vi "FPGA_Looped_PC.vi"() -> (0 "Chassis Temp History":i16[](array[numeric]), 3 "Chassis Temperature":i16)   [LabVIEW 2020]
uses:
  UIcontrol.ctl
  <vilib>/rvi/interface/RandomDataEmulation/nirviRandomDataOpen.vi
  <vilib>/rvi/interface/common/niFpgaCacheSessionInfoDynamic.vi
  <vilib>/Utility/error.llb/Error Cluster From Error Code.vi
  <vilib>/rvi/errors/niLvFpgaAdjustHostInterfaceError.vi
  <vilib>/rvi/interface/nirviOpenFPGA/nirviOpenFPGA.xnode
  FPGA_Temp.vi
  <vilib>/rvi/interface/nirviReadWriteControl/nirviReadWriteControl.xnode
  NiFpgaLv.dll
  <vilib>/rvi/interface/Simulation/niFpgaSimulationCallBeginRW.vi
panel:
  in  "cRIO Shutdown":bool
  in  "cRIO Save Data":bool
  in  "cRIO Start":bool
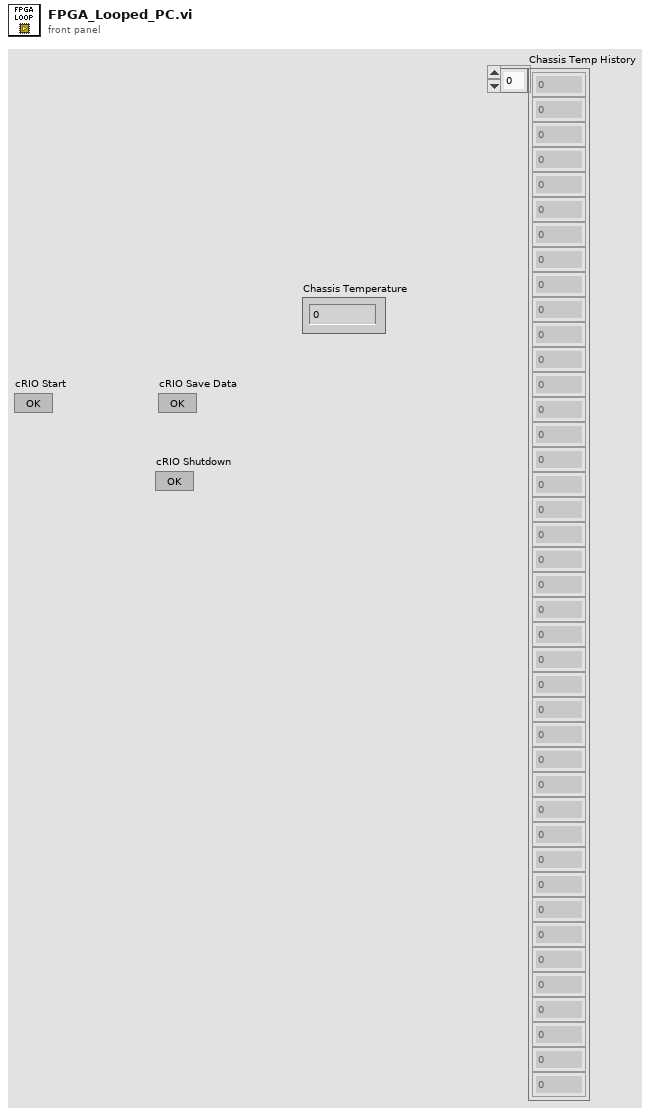
[diagram p1: front panel]
types:
  T1 = typedef "UIcontrol.ctl" = enum16{"Start", "Save Data", "Shutdown"}
  T2 = enum16{"open", "replace", "create", "open or create", "replace or create", "replace or create with confirmation"}
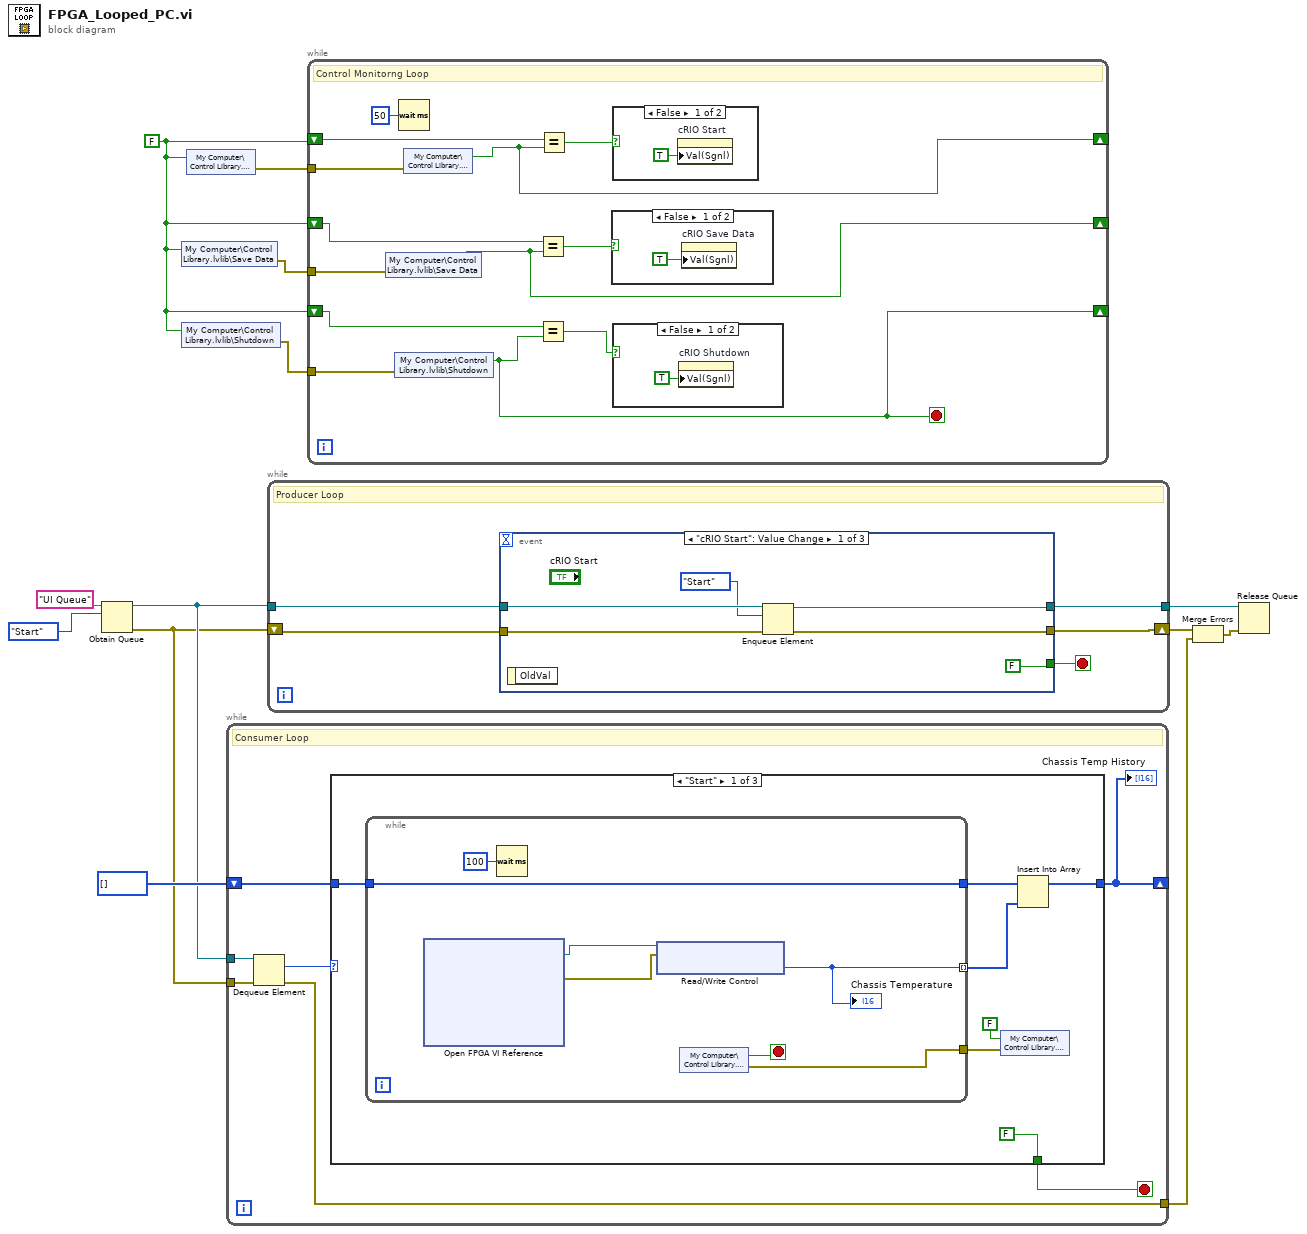
[diagram p0: block diagram]
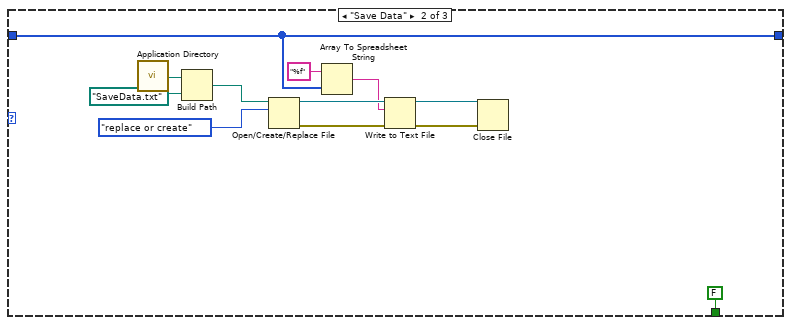
[diagram p5: hidden frame]
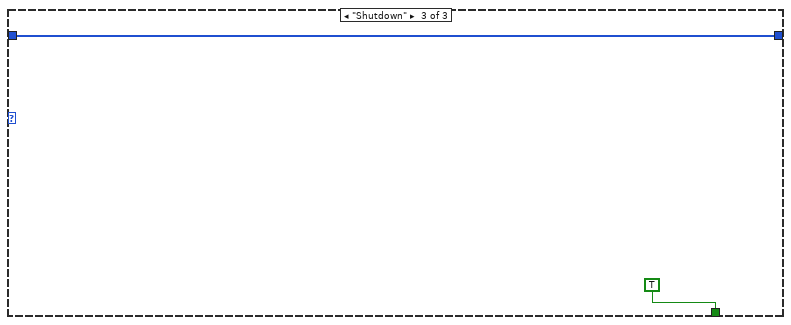
[diagram p6: hidden frame]
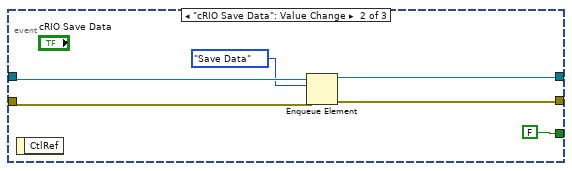
[diagram p7: hidden frame]
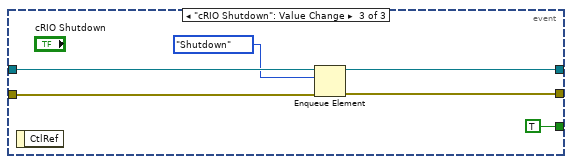
[diagram p8: hidden frame]
diagram:
  w4 = FALSE
  n1 = Obtain Queue(name (unnamed)="UI Queue", element data type=UIcontrol."Start") -> (queue out=w6:refnum<queue>, error out=w5:errorcluster)  [unwired: 3 in, 1 out]
  n2 = shared-variable "My Computer\\Control Library.lvlib\\Save Data"(w4) -> (error out=w2:errorcluster)  [unwired: 1 in]
  n3 = shared-variable "My Computer\\Control Library.lvlib\\Shutdown"(w4) -> (error out=w3:errorcluster)  [unwired: 1 in]
  n4 = shared-variable "My Computer\\Control Library.lvlib\\Start"(w4) -> (error out=w1:errorcluster)  [unwired: 1 in]
  n5 = while {
    tunnel: w6 -> [w20]
    tunnel: w5 -> [w19]
    tunnel: [w16] -> w8
    shift-right: [w15] -> _
    shift-left: i16[] [] -> [w14]
    stop <- w17 stop-if-true
    # "Consumer Loop"
    n6 = Dequeue Element(queue=w20, error in (no error)=w19) -> (element=w18:T1, error out=w16:errorcluster)  [unwired: 1 in, 2 out]
    n7 = case shown="\"Start\"" w18 {
      tunnel: [FALSE FALSE TRUE] -> w17
      tunnel: [w24 w45 w47] -> w15
      tunnel: w14 -> [w26 w45 w47]
      frame "Start" {
        n8 = while {
          tunnel: [w32] -> w25 mode=indexing
          tunnel: w26 -> [w30]
          tunnel: [w30] -> w23
          tunnel: [w28] -> w21
          stop <- w29 stop-if-true
          n9 = xnode "Open FPGA VI Reference"() -> ("FPGA VI Reference Out"=w34:refnum<k20>, "error out"=w33:errorcluster)  [unwired: 2 in]
          n10 = Wait (ms)(milliseconds to wait=u32 100) -> ()  [unwired: 1 out]
          n11 = xnode "Read/Write Control"("FPGA VI Reference In"=w34, "error in"=w33) -> ("Chassis Temperature"=w32:i16)  [unwired: 2 out]
          "Chassis Temperature" <- w32
          n12 = shared-variable "My Computer\\Control Library.lvlib\\Stop"() -> (w29:bool, error out=w28:errorcluster)  [unwired: 1 in]
        }
        n13 = shared-variable "My Computer\\Control Library.lvlib\\Stop"(FALSE ("Stop"), error in=w21) -> ()  [unwired: 1 out]
        n14 = Insert Into Array(array=w23, new element=w25) -> (w24:i16[])  [unwired: 1 in]
      }
      frame "Save Data" {
        n15 = call <vilib>:"Application Directory.vi"() -> ("Application Directory"=w38:path)
        n16 = Build Path(base path=w38, name or relative path=path "SaveData.txt") -> (appended path=w36:path)
        n17 = Open/Create/Replace File(file path (use dialog)=w36, operation (0:open)=T2."replace or create") -> (refnum out=w43:refnum<file>, error out=w41:errorcluster)  [unwired: 4 in, 1 out]
        n18 = Array To Spreadsheet String(array=w45, 3:"%f" ("format string")) -> (spreadsheet string=w42:string)  [unwired: 1 in]
        n19 = Write to Text File(file (use dialog)=w43, text=w42, error in=w41) -> (refnum out=w40:refnum<file>, error out=w39:errorcluster)  [unwired: 1 in, 1 out]
        n20 = Close File(refnum=w40, error in=w39) -> ()  [unwired: 2 out]
      }
      frame "Shutdown" {
      }
    }
    "Chassis Temp History" <- w15
  }
  n21 = while {
    tunnel: w6 -> [w52]
    shift-right: [w50] -> w9
    shift-left: w5 -> [w51]
    tunnel: [w49] -> w11
    stop <- w53 stop-if-true
    # "Producer Loop"
    n22 = event shown="[0] \"cRIO Start\": Value Change" {
      selector: _ -> [_ _ _]
      dyn-events: _ -> [_ _ _]
      timeout: _ -> [_ _ _]
      tunnel: [FALSE FALSE TRUE] -> w53
      tunnel: w52 -> [w58 w65 w71]
      tunnel: w51 -> [w57 w63 w70]
      tunnel: [w55 w64 w69] -> w49
      tunnel: [w56 w62 w68] -> w50
      event "cRIO Start": Value Change {
        n23 = event-data() -> ()  [unwired: 1 in, 1 out]
        n24 = Enqueue Element(queue=w58, element=UIcontrol."Start", error in (no error)=w57) -> (queue out=w55:refnum<queue>, error out=w56:errorcluster)  [unwired: 1 in, 1 out]
      }
      event "cRIO Save Data": Value Change {
        n25 = event-data() -> ()  [unwired: 1 in, 1 out]
        n26 = Enqueue Element(queue=w65, element=UIcontrol."Save Data", error in (no error)=w63) -> (queue out=w64:refnum<queue>, error out=w62:errorcluster)  [unwired: 1 in, 1 out]
      }
      event "cRIO Shutdown": Value Change {
        n27 = event-data() -> ()  [unwired: 1 in, 1 out]
        n28 = Enqueue Element(queue=w71, element=UIcontrol."Shutdown", error in (no error)=w70) -> (queue out=w69:refnum<queue>, error out=w68:errorcluster)  [unwired: 1 in, 1 out]
      }
    }
  }
  n29 = while {
    shift-right: [w80] -> _
    shift-left: w4 -> [w79]
    shift-right: [w78] -> _
    shift-left: w4 -> [w77]
    shift-right: [w76] -> _
    shift-left: w4 -> [w75]
    tunnel: w3 -> [w74]
    tunnel: w2 -> [w73]
    tunnel: w1 -> [w72]
    stop <- w80 stop-if-true
    # "Control Monitorng Loop"
    n30 = shared-variable "My Computer\\Control Library.lvlib\\Save Data"(error in=w73) -> (w78:bool)  [unwired: 1 out]
    n31 = shared-variable "My Computer\\Control Library.lvlib\\Shutdown"(error in=w74) -> (w80:bool)  [unwired: 1 out]
    n32 = Wait (ms)(milliseconds to wait=u32 50) -> ()  [unwired: 1 out]
    n33 = shared-variable "My Computer\\Control Library.lvlib\\Start"(error in=w72) -> (w76:bool)  [unwired: 1 out]
    n34 = Equal?(x=w77, y=w78) -> (x = y?=w83:bool)
    n35 = Equal?(x=w79, y=w80) -> (x = y?=w82:bool)
    n36 = Equal?(x=w75, y=w76) -> (x = y?=w84:bool)
    n37 = case shown="False" w83 {
      frame False {
        n38 = property on="cRIO Save Data" class="Bool (strict)"("Val(Sgnl)"=TRUE ("Value (Signaling)")) -> ()  [unwired: 2 in, 2 out]
      }
      frame True {
      }
    }
    n39 = case shown="False" w84 {
      frame False {
        n40 = property on="cRIO Start" class="Bool (strict)"("Val(Sgnl)"=TRUE ("Value (Signaling)")) -> ()  [unwired: 2 in, 2 out]
      }
      frame True {
      }
    }
    n41 = case shown="False" w82 {
      frame False {
        n42 = property on="cRIO Shutdown" class="Bool (strict)"("Val(Sgnl)"=TRUE ("Value (Signaling)")) -> ()  [unwired: 2 in, 2 out]
      }
      frame True {
      }
    }
  }
  n43 = Merge Errors(w9, w8) -> (w10:errorcluster)
  n44 = Release Queue(queue=w11, error in (no error)=w10) -> ()  [unwired: 1 in, 3 out]
